vi "Truck1.vi"(10 "Interior cargo capacity":dbl=67.0, 11 "Bed cargo capacity":dbl=64.4) -> (3 "truck":refnum<class "Truck.lvclass">)   [LabVIEW 2011]
doc: "Create and initialize a truck."
uses:
  Truck/Truck.lvclass
panel:
  in  "model":string="pickup"
  in  "make":string="Company B"
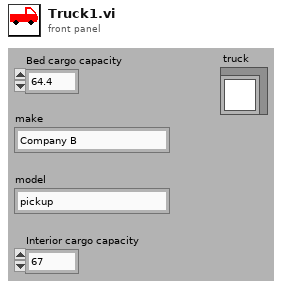
[diagram p1: front panel]
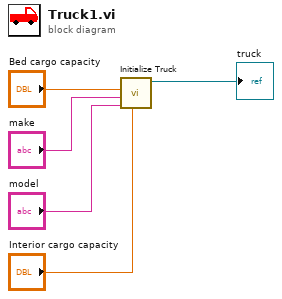
[diagram p0: block diagram]
diagram:
  n1 = call "Initialize Truck.vi"("Interior cargo capacity"="Interior cargo capacity", "model"="model", "make"="make", "Bed cargo capacity"="Bed cargo capacity") -> ("truck out"=→"truck":refnum<class "Truck.lvclass">)  [unwired: 7 in]
